vi "lineare_a_tratti(SubVI).vi"(0 "image in":T2, 1 "soglia in":i32, 2 "pendenza 1":dbl, 5 "soglia 1":i32, 7 "pendenza in":dbl, 11 "error in (no error)":errorcluster) -> (3 "Waveform Graph":i32[](graph), 8 "Output":T2(plugin-control), 10 "Array":i32[](array[numeric]), 15 "error out":errorcluster)   [LabVIEW 2020]
uses:
  <vilib>/vision/Image Controls.llb/IMAQ Image.ctl
  <vilib>/vision/NI_Vision_Development_Module.lvlib
panel:
  out "Input Histohraph 2":T1(graph)
  out "Input cumulative histogram 2":u32[](graph)
  out "Input":T2(plugin-control)
  out "Output Histohraph":T1(graph)
  out "Output cumulative histogram":u32[](graph)
  in  "image Dst":T2
  in  "stop":bool
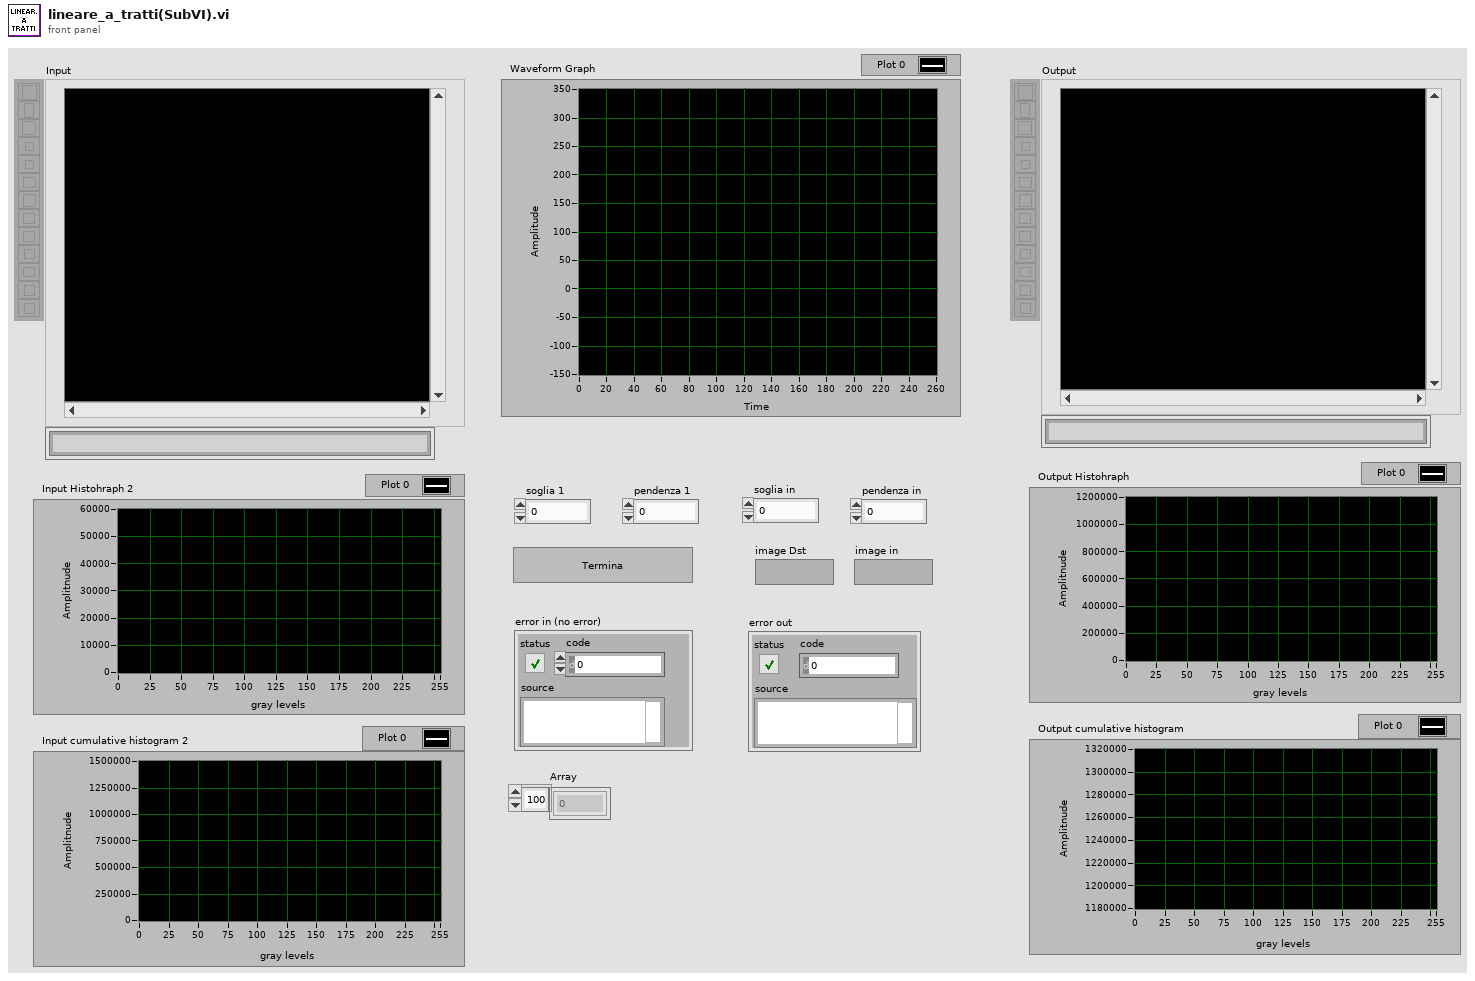
[diagram p1: front panel]
types:
  T1 = cluster{"Starting Value":sgl, "Incremental Value":sgl, "Histogram":u32[]}
  T2 = typedef "IMAQ Image.ctl" = refnum<image>
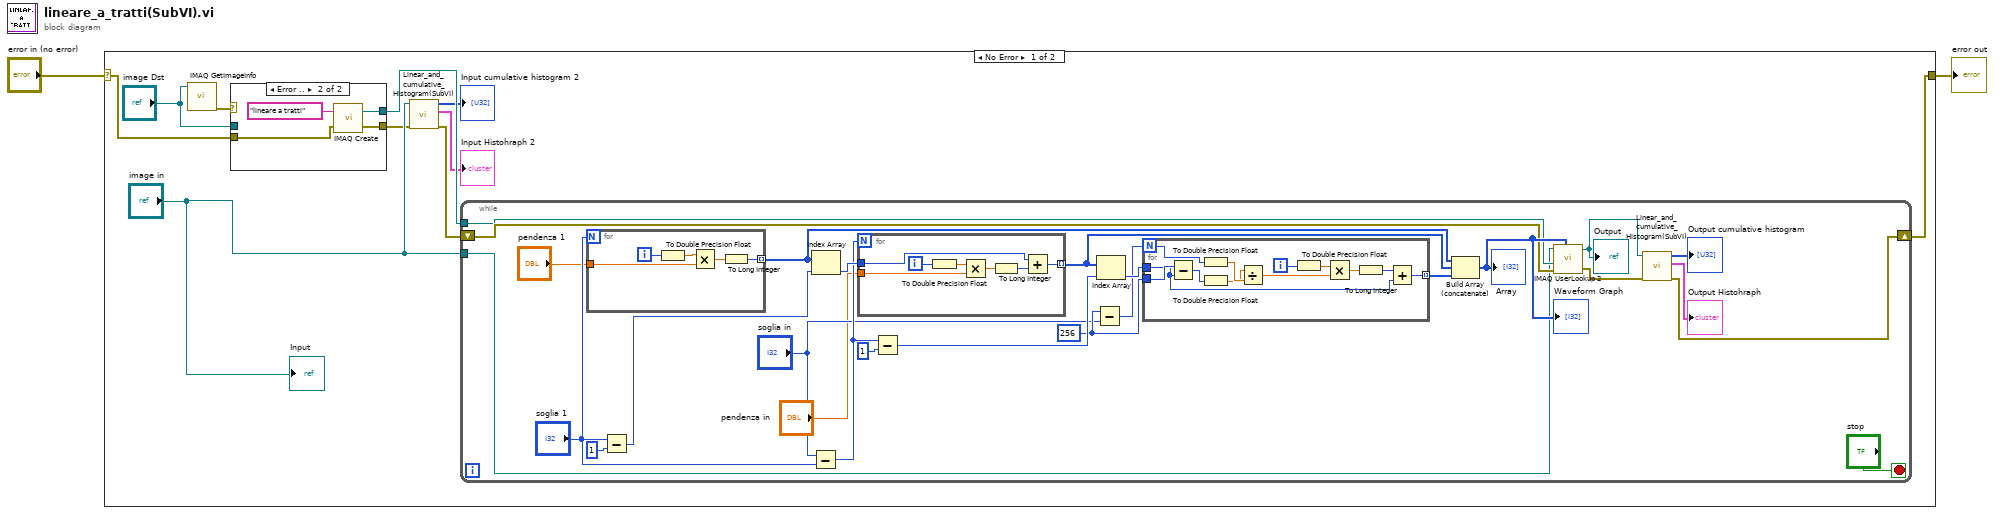
[diagram p0: block diagram]
diagram:
  n1 = case shown="No Error" "error in (no error)" {
    selector: "error in (no error)" -> [w4 w69]
    tunnel: [w12 w69] -> w2
    frame No Error {
      n2 = call "IMAQ GetImageInfo"("Image"="image Dst") -> ("error out"=w10:errorcluster)  [unwired: 3 in, 7 out]
      n3 = case shown="Error .." w10 {
        tunnel: [w14 w16] -> w9
        tunnel: "image Dst" -> [w14 _]
        tunnel: [w13 w18] -> w3
        tunnel: w4 -> [w13 w15]
        frame No Error {
        }
        frame Error {
          n4 = call "IMAQ Create"("Image Name"="lineare a tratti", "error in (no error)"=w15) -> ("New Image"=w16:T2, "error out"=w18:errorcluster)  [unwired: 3 in]
        }
      }
      n5 = call "Linear_and_cumulative_Histogram(SubVI).vi"("error in (no error)"=w3, "Image GRAY"="image in") -> ("error out"=w6:errorcluster, "Linear Histogram"=→"Input Histohraph 2":T1, "Cumulative Histogram"=→"Input cumulative histogram 2":u32[])  [unwired: 7 in]
      n6 = while {
        shift-right: [w23] -> w12
        shift-left: w6 -> [w27]
        tunnel: w9 -> [w20]
        tunnel: "image in" -> [w19]
        stop <- "stop" stop-if-true
        w32 = 256 ("x")
        n7 = for {
          N: "soglia 1" -> [_]
          tunnel: "pendenza 1" -> [w68]
          tunnel: [w64] -> w40 mode=indexing
          i -> [w66]
          n8 = To Double Precision Float(number=w66) -> (double precision float=w67:dbl)
          n9 = Multiply(x=w67, y=w68) -> (x*y=w65:dbl)
          n10 = To Long Integer(number=w65) -> (32bit integer=w64:i32)
        }
        n11 = Subtract(x="soglia 1", y=1) -> (x-y=w43:i32)
        n12 = Subtract(x="soglia in", y="soglia 1") -> (x-y=w34:i32)
        n13 = Index Array(array=w40, index=w43) -> (element=w44:i32)
        n14 = for {
          N: w34 -> [_]
          tunnel: "pendenza in" -> [w63]
          tunnel: [w58] -> w37 mode=indexing
          tunnel: w44 -> [w59]
          i -> [w57]
          n15 = To Double Precision Float(number=w57) -> (double precision float=w62:dbl)
          n16 = Multiply(x=w62, y=w63) -> (x*y=w61:dbl)
          n17 = To Long Integer(number=w61) -> (32bit integer=w60:i32)
          n18 = Add(x=w59, y=w60) -> (x+y=w58:i32)
        }
        n19 = Subtract(x=w34, y=1) -> (x-y=w36:i32)
        n20 = Subtract(x=w32, y="soglia in") -> (x-y=w30:i32)
        n21 = Index Array(array=w37, index=w36) -> (element=w33:i32)
        n22 = for {
          N: w30 -> [w54]
          tunnel: w32 -> [w55]
          tunnel: w33 -> [w50]
          tunnel: [w48] -> w38 mode=indexing
          i -> [w47]
          n23 = Subtract(x=w55, y=w50) -> (x-y=w51:i32)
          n24 = To Double Precision Float(number=w54) -> (double precision float=w46:dbl)
          n25 = To Double Precision Float(number=w51) -> (double precision float=w45:dbl)
          n26 = Divide(x=w45, y=w46) -> (x/y=w56:dbl)
          n27 = To Double Precision Float(number=w47) -> (double precision float=w53:dbl)
          n28 = Multiply(x=w53, y=w56) -> (x*y=w52:dbl)
          n29 = To Long Integer(number=w52) -> (32bit integer=w49:i32)
          n30 = Add(x=w49, y=w50) -> (x+y=w48:i32)
        }
        n31 = Build Array (concatenate)(w40, w37, w38) -> (w39:i32[])
        "Waveform Graph" <- w39
        "Array" <- w39
        n32 = call "IMAQ UserLookup 2"("Image Src"=w19, "Lookup Table"=w39, "Image Dst"=w20, "error in (no error)"=w27) -> ("Image Dst Out"=w25:T2, "error out"=w24:errorcluster)  [unwired: 3 in]
        "Output" <- w25
        n33 = call "Linear_and_cumulative_Histogram(SubVI).vi"("error in (no error)"=w24, "Image GRAY"=w25) -> ("error out"=w23:errorcluster, "Linear Histogram"=→"Output Histohraph":T1, "Cumulative Histogram"=→"Output cumulative histogram":u32[])  [unwired: 7 in]
      }
      "Input" <- "image in"
    }
    frame Error {
    }
  }
  "error out" <- w2
